vi "Populate Recorder List.vi"(4 "Seconds between samples":dbl=1.0 format="%_4f", 8 "error in (no error)":errorcluster, 11 "VISA Resourse Names":refnum<visa-resource-name>[](array[refnum])) -> (0 "error out":errorcluster, 2 "Names":string[](array[string]), 3 "Instrument List":refnum<class "Instrument Actor.lvclass">[](array[class]))   [LabVIEW 2019]
uses:
  Instrument Actor/Instrument Actor.lvclass
  NHMFL_Core/Libraries/Instruments/Device/Device type.ctl
  Temperature Controller/Temperature Controller.lvclass
  C:/GitHub/LabActor/Instrument Actor/Instrument Actor.lvclass
  NHMFL_Core/Libraries/Instruments/Cryo-con/Cryo-Con Driver/Cryo-Con Driver.lvclass
  C:/GitHub/NHMFL_Core/Libraries/Instruments/VISA Instrument/VISA Instrument.lvclass
  C:/GitHub/NHMFL_Core/Libraries/Instruments/Instrument Driver/Instrument Driver.lvclass
  C:/GitHub/NHMFL_Core/Libraries/Instruments/Temperature Controller Driver/Temperature Controller Driver.lvclass
  NHMFL_Core/Libraries/Instruments/VISA Instrument/VISA Instrument.lvclass/VISA Instrument.ctl
  NHMFL_Core/Libraries/Instruments/Instrument Driver/Instrument Driver.lvclass/Instrument Driver.ctl
  NHMFL_Core/Libraries/Instruments/Neocera/Neocera Driver/Neocera Driver.lvclass
  NHMFL_Core/Libraries/Instruments/LakeShore/LakeShore T Controller Driver/LakeShore T Controller Driver.lvclass
  NHMFL_Core/Libraries/Instruments/Arduino Temperature Controller/Arduino Temperature Controller Driver/Arduino Temperature Controller Driver.lvclass
  Channel Scanner/Channel Scanner.lvclass
  NHMFL_Core/Libraries/Instruments/LR-700/LR-700 Driver/LR-700 Driver.lvclass
  Instrument Actor/Instrument Actor.lvclass/Instrument Actor.ctl
  NHMFL_Core/Libraries/Instruments/Fluke/Fluke 1586A Driver.lvclass
  Fluke/Fluke Recorder.lvclass
  NHMFL_Core/Libraries/Instruments/Oxford/Oxford PS Driver/Oxford PS Driver.lvclass
  NHMFL_Core/Libraries/Instruments/AH/Andeen-Hagerling Driver/Andeen-Hagerling Driver.lvclass
  NHMFL_Core/Libraries/Instruments/Keithley/Keithley Driver/Keithley Driver.lvclass
  Keithley/Keithley Recorder.lvclass
  NHMFL_Core/Libraries/Instruments/Keithley/Keithley Driver/Keithley Driver.lvclass/Keithley Driver.ctl
  NHMFL_Core/Libraries/Instruments/LakeShore/LakeShore 370 Driver/LakeShore 370 Driver.lvclass
  NHMFL_Core/Libraries/Instruments/SRS/SRS Lockin Driver/SRS Lockin Driver.lvclass
  NHMFL_Core/Libraries/Instruments/HP/HP Counter Driver/HP Counter Driver.lvclass
  NHMFL_Core/Libraries/Instruments/Oxford/IPS120/IPS120.lvclass
  Sweeper/Sweeper.lvclass
  NHMFL_Core/Libraries/Instruments/Oxford/ITC503/ITC-503 Driver.lvclass
  NHMFL_Core/Libraries/Instruments/VISA Instrument/Write VISA resource.vi
  NHMFL_Core/Libraries/Instruments/Instrument Driver/Write Recorder name.vi
  Instrument Actor/Write Instrument driver.vi
  NHMFL_Core/Libraries/Instruments/Keithley/Keithley Driver/Write Source-meter.vi
  NHMFL_Core/Libraries/Instruments/Keithley/Keithley Driver/Write Auto-init.vi
  Temperature Controller/Write T ctl driver.vi
panel:
  in  "Instrument":T1=enum."LkShr 340 chA&B"
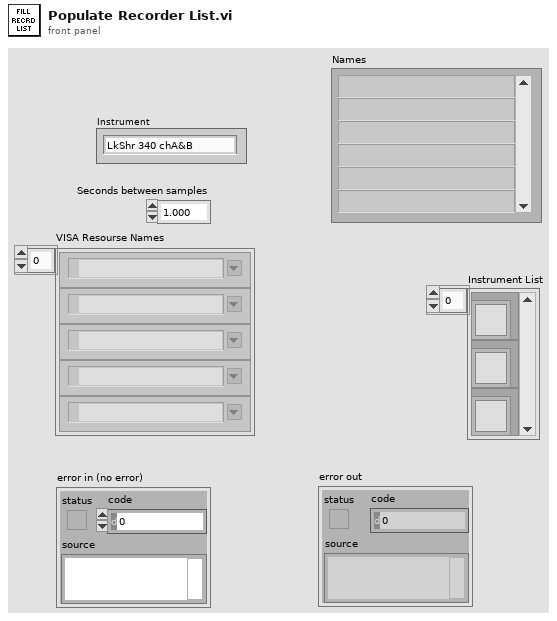
[diagram p1: front panel]
types:
  T1 = typedef "Device type.ctl" = enum16{"NONE", "Neocera 21", "LakeShore 335", "LakeShore 336", "LakeShore 340", "LkShr 340 chA&B", "LakeShore 370", "SRS 850", "SRS 830", "LR 700", "EG&G 5302", "EG&G 7260", "EG&G 7280", "AH 2500", "AH 2550", "AH 2700", "Keithley meter", "Keithley electrometer", "Keithley 182", "HP 5385", "HP 53181", "HP 53132", "ITC503", "IPS120", "Oxford Mercury IPS", "Oxford PS", "Test", "DC Facility Magnet", "Cryomagnetics PS", "Keithley 2400", "Keithley current source", "Cryo-Con 22C", "HP87NN", "HP4395A", "Agilent 34410A", "Arduino TC", "Cryo-Con 54", "Fluke 1586A"}
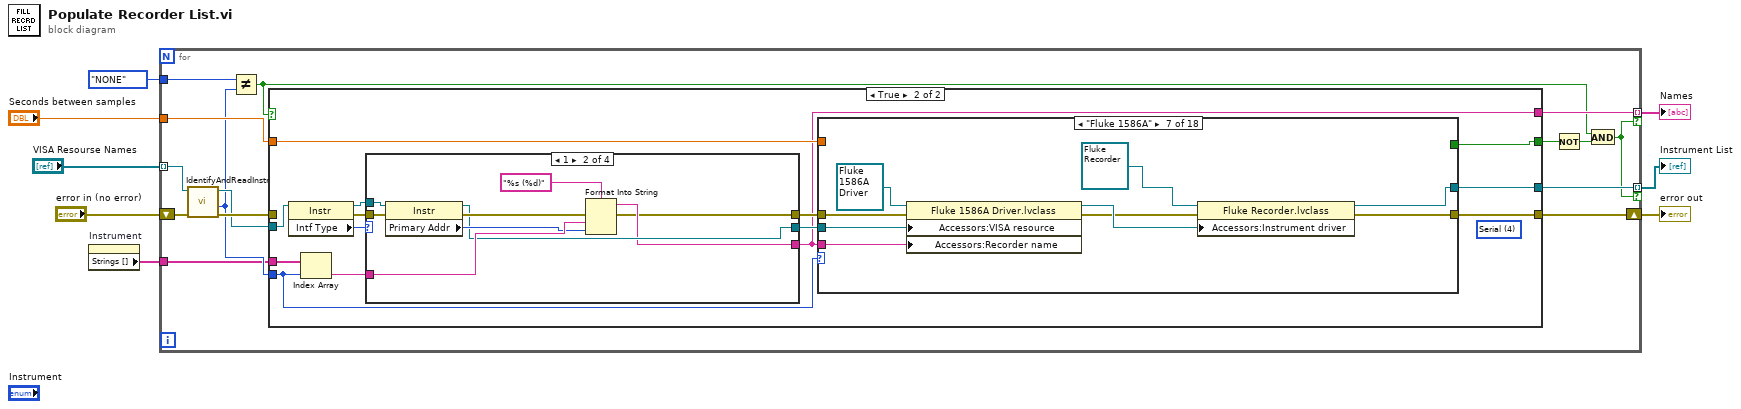
[diagram p0: block diagram]
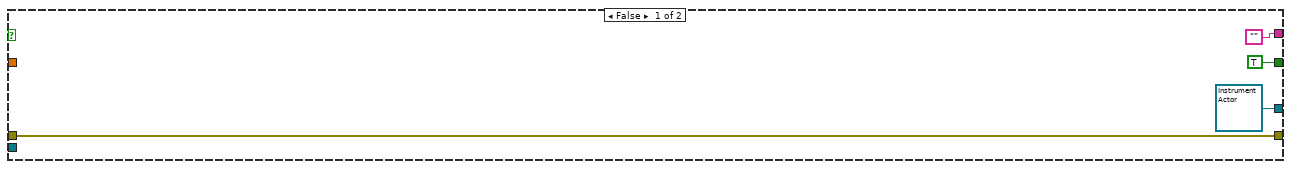
[diagram p2: hidden frame]
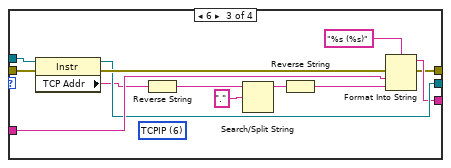
[diagram p4: hidden frame]
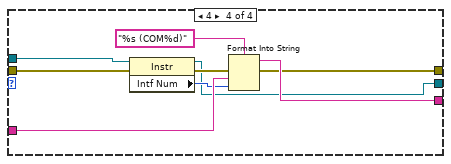
[diagram p5: hidden frame]
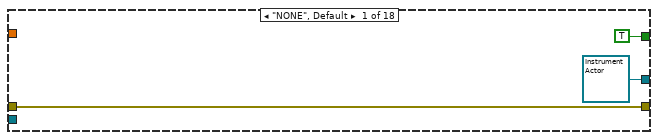
[diagram p6: hidden frame]
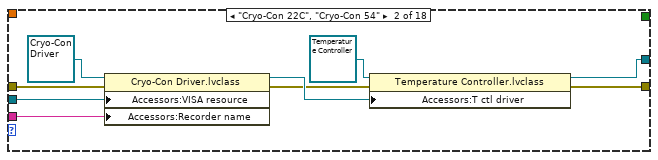
[diagram p7: hidden frame]
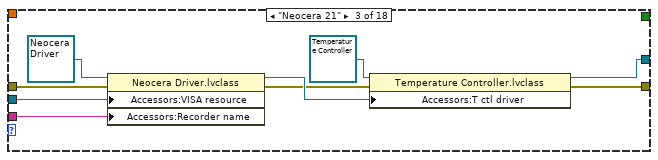
[diagram p8: hidden frame]
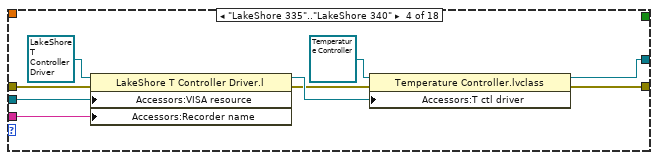
[diagram p9: hidden frame]
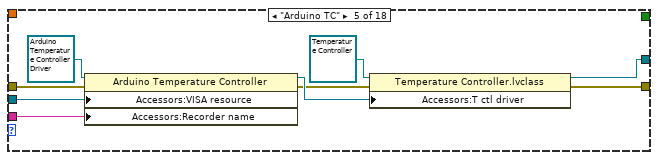
[diagram p10: hidden frame]
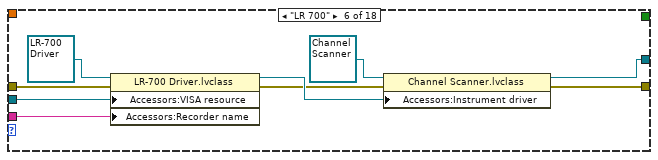
[diagram p11: hidden frame]
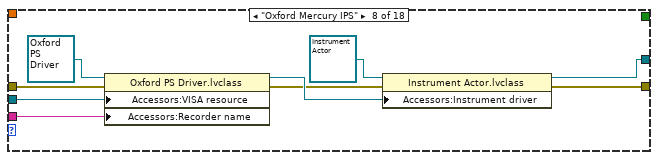
[diagram p12: hidden frame]
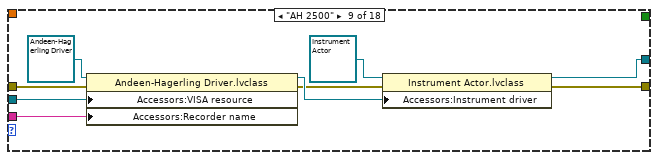
[diagram p13: hidden frame]
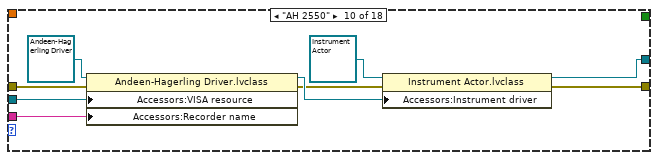
[diagram p14: hidden frame]
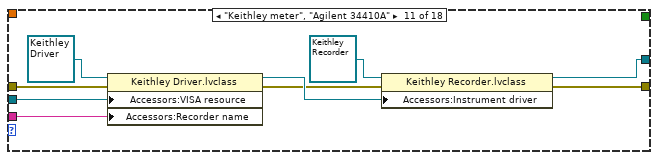
[diagram p15: hidden frame]
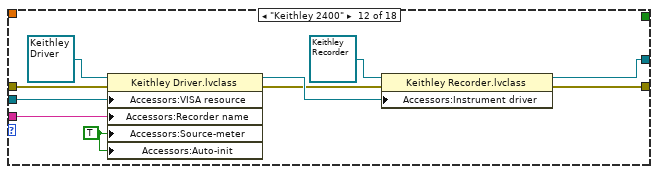
[diagram p16: hidden frame]
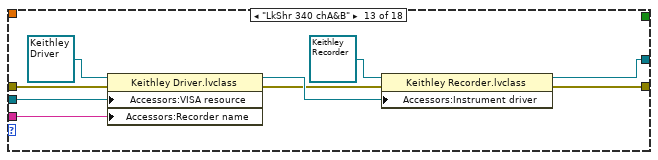
[diagram p17: hidden frame]
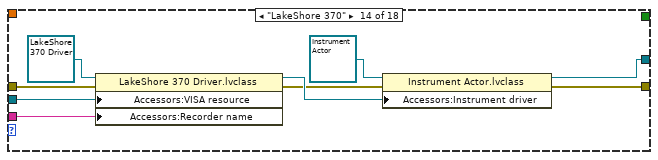
[diagram p18: hidden frame]
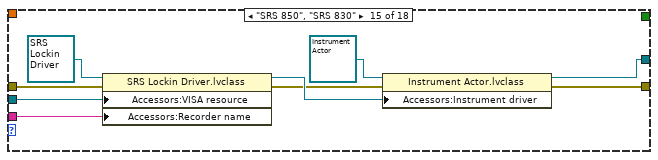
[diagram p19: hidden frame]
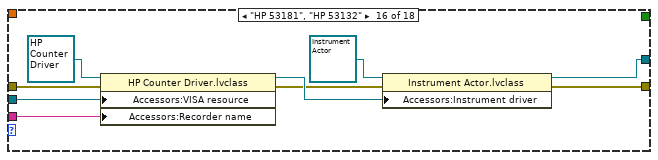
[diagram p20: hidden frame]
diagram:
  n1 = property on="Instrument" class="Enum (strict)"() -> ("Strings []"=w4:string[])  [unwired: 2 in, 2 out]
  n2 = for {
    tunnel: "VISA Resourse Names" -> [w21] mode=indexing
    shift-right: [w18] -> w6
    shift-left: "error in (no error)" -> [w23]
    tunnel: "Seconds between samples" -> [w20]
    tunnel: w4 -> [w15]
    tunnel: Device_type."NONE" ("Instrument") -> [w17]
    tunnel: [w14] -> w2 mode=indexing if=w11
    tunnel: [w13] -> w1 mode=indexing if=w11
    n3 = call "IdentifyAndReadInstr.vi"("error in (no error)"=w23, "VISA Resource Name"=w21) -> ("error out"=w22:errorcluster, "Instrument"=w16:T1, "VISA Resource Name Out"=w19:refnum<visa-resource-name>)  [unwired: 6 in, 1 out]
    n4 = Not Equal?(x=w17, y=w16) -> (x != y?=w12:bool)
    n5 = case shown="True" w12 {
      tunnel: w22 -> [w27 _]
      tunnel: w20 -> [_ w41]
      tunnel: w19 -> [_ w36]
      tunnel: w16 -> [_ w38]
      tunnel: [refnum<class "Instrument Actor.lvclass"> refnum ("Instrument Recorder.lvclass") w33] -> w14
      tunnel: [w27 w30] -> w18
      tunnel: w15 -> [_ w40]
      tunnel: ["" w29] -> w13
      tunnel: [TRUE w28] -> w10
      frame False {
      }
      frame True {
        (unwired) u16 4 items=["GPIB"=1, "VXI"=2, "GPIB-VXI"=3, "Serial"=4, "PXI"=5, "TCPIP"=6, "USB"=7, "FireWire"=9] ("Interface Information:Interface Type")
        n6 = property class="Instr"(reference=w36) -> (reference out=w37:refnum<visa-resource-name>, error out=w35:errorcluster, "Intf Type"=w34:u16)  [unwired: 1 in]
        n7 = Index Array(array=w40, index=w38) -> (element=w39:string)
        n8 = case shown="1" w34 {
          tunnel: w39 -> [w42 w51 w64 w73]
          tunnel: [w43 w49 w63 w67] -> w31
          tunnel: [w42 w48 w62 w71] -> w29
          tunnel: [w44 w47 w61 w70] -> w32
          tunnel: w37 -> [w43 w46 w60 w69]
          tunnel: w35 -> [w44 w45 w59 w68]
          frame 0, Default {
          }
          frame 1 {
            n9 = property class="Instr"(reference=w46, error in=w45) -> (reference out=w49:refnum<visa-resource-name>, error out=w53:errorcluster, "Primary Addr"=w50:u16)
            n10 = Format Into String(format string="%s (%d)", error in=w53, w51, w50) -> (resulting string=w48:string, error out=w47:errorcluster)  [unwired: 1 in]
          }
          frame 6 {
            (unwired) u16 6 items=["GPIB"=1, "VXI"=2, "GPIB-VXI"=3, "Serial"=4, "PXI"=5, "TCPIP"=6, "USB"=7, "FireWire"=9] ("Interface Information:Interface Type")
            n11 = property class="Instr"(reference=w60, error in=w59) -> (reference out=w63:refnum<visa-resource-name>, error out=w66:errorcluster, "TCP Addr"=w58:string)
            n12 = Reverse String(1:w58) -> (0:w56:string)
            n13 = Search/Split String(string=w56, search string/char (-)="." ("regular expression")) -> (substring before match=w55:string)  [unwired: 1 in, 2 out]
            n14 = Reverse String(1:w55) -> (0:w57:string)
            n15 = Format Into String(format string="%s (%s)", error in=w66, w64, w57) -> (resulting string=w62:string, error out=w61:errorcluster)  [unwired: 1 in]
          }
          frame 4 {
            n16 = property class="Instr"(reference=w69, error in=w68) -> (reference out=w67:refnum<visa-resource-name>, error out=w75:errorcluster, "Intf Num"=w72:u16)
            n17 = Format Into String(format string="%s (COM%d)", error in=w75, w73, w72) -> (resulting string=w71:string, error out=w70:errorcluster)  [unwired: 1 in]
          }
        }
        n18 = case shown="\"Fluke 1586A\"" w38 {
          tunnel: w32 -> [w78 w81 w90 w99 w108 w117 w127 w136 w145 w154 w163 w173 w182 w191 w200 w209 w219 w228]
          tunnel: [w78 w80 w89 w98 w107 w116 w126 w135 w144 w153 w162 w172 w181 w190 w199 w208 w218 w227] -> w30
          tunnel: [refnum<class "Instrument Actor.lvclass"> refnum ("Instrument Recorder.lvclass") w86 w95 w104 w113 w119 w129 w138 w147 w156 w165 w175 w184 w193 w202 w211 w221 w230] -> w33
          tunnel: w41 -> [_ _ _ _ _ _ _ _ _ _ _ _ _ _ _ _ _ _]
          tunnel: w31 -> [_ w83 w92 w101 w110 w121 w130 w139 w148 w157 w166 w176 w185 w194 w203 w212 w222 w231]
          tunnel: w29 -> [_ w79 w88 w97 w106 w115 w125 w134 w143 w152 w161 w171 w180 w189 w198 w207 w217 w226]
          tunnel: [TRUE _ _ _ _ _ _ _ _ _ _ _ _ _ _ _ _ _] -> w28
          frame "NONE", Default {
          }
          frame "Cryo-Con 22C", "Cryo-Con 54" {
            n19 = property class="Cryo-Con Driver.lvclass"(reference=refnum<class "Cryo-Con Driver.lvclass"> refnum ("Cryo-Con Driver.lvclass"), error in=w81, "Accessors:VISA resource"=w83, "Accessors:Recorder name"=w79) -> (reference out=w84:refnum<class "Cryo-Con Driver.lvclass">, error out=w82:errorcluster)
            n20 = property class="Temperature Controller.lvclass"(reference=refnum<class "Temperature Controller.lvclass"> refnum ("Temperature Controller.lvclass"), error in=w82, "Accessors:T ctl driver"=w84) -> (reference out=w86:refnum<class "Temperature Controller.lvclass">, error out=w80:errorcluster)
          }
          frame "Neocera 21" {
            n21 = property class="Neocera Driver.lvclass"(reference=refnum<class "Neocera Driver.lvclass"> refnum ("Neocera Driver.lvclass"), error in=w90, "Accessors:VISA resource"=w92, "Accessors:Recorder name"=w88) -> (reference out=w93:refnum<class "Neocera Driver.lvclass">, error out=w91:errorcluster)
            n22 = property class="Temperature Controller.lvclass"(reference=refnum<class "Temperature Controller.lvclass"> refnum ("Temperature Controller.lvclass"), error in=w91, "Accessors:T ctl driver"=w93) -> (reference out=w95:refnum<class "Temperature Controller.lvclass">, error out=w89:errorcluster)
          }
          frame "LakeShore 335".."LakeShore 340" {
            n23 = property class="LakeShore T Controller Driver.l"(reference=refnum<class "LakeShore T Controller Driver.lvclass"> refnum ("LakeShore T Controller Driver.lvclass"), error in=w99, "Accessors:VISA resource"=w101, "Accessors:Recorder name"=w97) -> (reference out=w102:refnum<class "LakeShore T Controller Driver.lvclass">, error out=w100:errorcluster)
            n24 = property class="Temperature Controller.lvclass"(reference=refnum<class "Temperature Controller.lvclass"> refnum ("Temperature Controller.lvclass"), error in=w100, "Accessors:T ctl driver"=w102) -> (reference out=w104:refnum<class "Temperature Controller.lvclass">, error out=w98:errorcluster)
          }
          frame "Arduino TC" {
            n25 = property class="Arduino Temperature Controller "(reference=refnum<class "Arduino Temperature Controller Driver.lvclass"> refnum ("Arduino Temperature Controller Driver.lvclass"), error in=w108, "Accessors:VISA resource"=w110, "Accessors:Recorder name"=w106) -> (reference out=w111:refnum<class "Arduino Temperature Controller Driver.lvclass">, error out=w109:errorcluster)
            n26 = property class="Temperature Controller.lvclass"(reference=refnum<class "Temperature Controller.lvclass"> refnum ("Temperature Controller.lvclass"), error in=w109, "Accessors:T ctl driver"=w111) -> (reference out=w113:refnum<class "Temperature Controller.lvclass">, error out=w107:errorcluster)
          }
          frame "LR 700" {
            n27 = property class="LR-700 Driver.lvclass"(reference=refnum<class "LR-700 Driver.lvclass"> refnum ("LR-700 Driver.lvclass"), error in=w117, "Accessors:VISA resource"=w121, "Accessors:Recorder name"=w115) -> (reference out=w122:refnum<class "LR-700 Driver.lvclass">, error out=w118:errorcluster)
            n28 = property class="Channel Scanner.lvclass"(reference=refnum<class "Channel Scanner.lvclass"> refnum ("Channel Scanner.lvclass"), error in=w118, "Accessors:Instrument driver"=w122) -> (reference out=w119:refnum<class "Channel Scanner.lvclass">, error out=w116:errorcluster)
          }
          frame "Fluke 1586A" {
            n29 = property class="Fluke 1586A Driver.lvclass"(reference=refnum<class "Fluke 1586A Driver.lvclass"> refnum ("Fluke 1586A Driver.lvclass"), error in=w127, "Accessors:VISA resource"=w130, "Accessors:Recorder name"=w125) -> (reference out=w131:refnum<class "Fluke 1586A Driver.lvclass">, error out=w128:errorcluster)
            n30 = property class="Fluke Recorder.lvclass"(reference=refnum<class "Fluke Recorder.lvclass"> refnum ("Instrument Recorder.lvclass"), error in=w128, "Accessors:Instrument driver"=w131) -> (reference out=w129:refnum<class "Fluke Recorder.lvclass">, error out=w126:errorcluster)
          }
          frame "Oxford Mercury IPS" {
            n31 = property class="Oxford PS Driver.lvclass"(reference=refnum<class "Oxford PS Driver.lvclass"> refnum ("Oxford PS Driver.lvclass"), error in=w136, "Accessors:VISA resource"=w139, "Accessors:Recorder name"=w134) -> (reference out=w140:refnum<class "Oxford PS Driver.lvclass">, error out=w137:errorcluster)
            n32 = property class="Instrument Actor.lvclass"(reference=refnum<class "Instrument Actor.lvclass"> refnum ("Instrument Recorder.lvclass"), error in=w137, "Accessors:Instrument driver"=w140) -> (reference out=w138:refnum<class "Instrument Actor.lvclass">, error out=w135:errorcluster)
          }
          frame "AH 2500" {
            n33 = property class="Andeen-Hagerling Driver.lvclass"(reference=refnum<class "Andeen-Hagerling Driver.lvclass"> refnum ("Andeen-Hagerling Driver.lvclass"), error in=w145, "Accessors:VISA resource"=w148, "Accessors:Recorder name"=w143) -> (reference out=w149:refnum<class "Andeen-Hagerling Driver.lvclass">, error out=w146:errorcluster)
            n34 = property class="Instrument Actor.lvclass"(reference=refnum<class "Instrument Actor.lvclass"> refnum ("Instrument Recorder.lvclass"), error in=w146, "Accessors:Instrument driver"=w149) -> (reference out=w147:refnum<class "Instrument Actor.lvclass">, error out=w144:errorcluster)
          }
          frame "AH 2550" {
            n35 = property class="Andeen-Hagerling Driver.lvclass"(reference=refnum<class "Andeen-Hagerling Driver.lvclass"> refnum ("Andeen-Hagerling Driver.lvclass"), error in=w154, "Accessors:VISA resource"=w157, "Accessors:Recorder name"=w152) -> (reference out=w158:refnum<class "Andeen-Hagerling Driver.lvclass">, error out=w155:errorcluster)
            n36 = property class="Instrument Actor.lvclass"(reference=refnum<class "Instrument Actor.lvclass"> refnum ("Instrument Recorder.lvclass"), error in=w155, "Accessors:Instrument driver"=w158) -> (reference out=w156:refnum<class "Instrument Actor.lvclass">, error out=w153:errorcluster)
          }
          frame "Keithley meter", "Agilent 34410A" {
            n37 = property class="Keithley Driver.lvclass"(reference=refnum<class "Keithley Driver.lvclass"> refnum ("Keithley Driver.lvclass"), error in=w163, "Accessors:VISA resource"=w166, "Accessors:Recorder name"=w161) -> (reference out=w167:refnum<class "Keithley Driver.lvclass">, error out=w164:errorcluster)
            n38 = property class="Keithley Recorder.lvclass"(reference=refnum<class "Keithley Recorder.lvclass"> refnum ("Instrument Recorder.lvclass"), error in=w164, "Accessors:Instrument driver"=w167) -> (reference out=w165:refnum<class "Keithley Recorder.lvclass">, error out=w162:errorcluster)
          }
          frame "Keithley 2400" {
            w169 = TRUE ("Source-meter")
            n39 = property class="Keithley Driver.lvclass"(reference=refnum<class "Keithley Driver.lvclass"> refnum ("Keithley Driver.lvclass"), error in=w173, "Accessors:VISA resource"=w176, "Accessors:Recorder name"=w171, "Accessors:Source-meter"=w169, "Accessors:Auto-init"=w169) -> (reference out=w177:refnum<class "Keithley Driver.lvclass">, error out=w174:errorcluster)
            n40 = property class="Keithley Recorder.lvclass"(reference=refnum<class "Keithley Recorder.lvclass"> refnum ("Instrument Recorder.lvclass"), error in=w174, "Accessors:Instrument driver"=w177) -> (reference out=w175:refnum<class "Keithley Recorder.lvclass">, error out=w172:errorcluster)
          }
          frame "LkShr 340 chA&B" {
            n41 = property class="Keithley Driver.lvclass"(reference=refnum<class "Keithley Driver.lvclass"> refnum ("Keithley Driver.lvclass"), error in=w182, "Accessors:VISA resource"=w185, "Accessors:Recorder name"=w180) -> (reference out=w186:refnum<class "Keithley Driver.lvclass">, error out=w183:errorcluster)
            n42 = property class="Keithley Recorder.lvclass"(reference=refnum<class "Keithley Recorder.lvclass"> refnum ("Instrument Recorder.lvclass"), error in=w183, "Accessors:Instrument driver"=w186) -> (reference out=w184:refnum<class "Keithley Recorder.lvclass">, error out=w181:errorcluster)
          }
          frame "LakeShore 370" {
            n43 = property class="LakeShore 370 Driver.lvclass"(reference=refnum<class "LakeShore 370 Driver.lvclass"> refnum ("LakeShore 370 Driver.lvclass"), error in=w191, "Accessors:VISA resource"=w194, "Accessors:Recorder name"=w189) -> (reference out=w195:refnum<class "LakeShore 370 Driver.lvclass">, error out=w192:errorcluster)
            n44 = property class="Instrument Actor.lvclass"(reference=refnum<class "Instrument Actor.lvclass"> refnum ("Instrument Recorder.lvclass"), error in=w192, "Accessors:Instrument driver"=w195) -> (reference out=w193:refnum<class "Instrument Actor.lvclass">, error out=w190:errorcluster)
          }
          frame "SRS 850", "SRS 830" {
            n45 = property class="SRS Lockin Driver.lvclass"(reference=refnum<class "SRS Lockin Driver.lvclass"> refnum ("SRS Lockin Driver.lvclass"), error in=w200, "Accessors:VISA resource"=w203, "Accessors:Recorder name"=w198) -> (reference out=w204:refnum<class "SRS Lockin Driver.lvclass">, error out=w201:errorcluster)
            n46 = property class="Instrument Actor.lvclass"(reference=refnum<class "Instrument Actor.lvclass"> refnum ("Instrument Recorder.lvclass"), error in=w201, "Accessors:Instrument driver"=w204) -> (reference out=w202:refnum<class "Instrument Actor.lvclass">, error out=w199:errorcluster)
          }
          frame "HP 53181", "HP 53132" {
            n47 = property class="HP Counter Driver.lvclass"(reference=refnum<class "HP Counter Driver.lvclass"> refnum ("HP Counter Driver.lvclass"), error in=w209, "Accessors:VISA resource"=w212, "Accessors:Recorder name"=w207) -> (reference out=w213:refnum<class "HP Counter Driver.lvclass">, error out=w210:errorcluster)
            n48 = property class="Instrument Actor.lvclass"(reference=refnum<class "Instrument Actor.lvclass"> refnum ("Instrument Recorder.lvclass"), error in=w210, "Accessors:Instrument driver"=w213) -> (reference out=w211:refnum<class "Instrument Actor.lvclass">, error out=w208:errorcluster)
          }
          frame "IPS120" {
            n49 = property class="IPS120.lvclass"(reference=refnum<class "IPS120.lvclass"> refnum ("IPS120.lvclass"), error in=w219, "Accessors:VISA resource"=w222, "Accessors:Recorder name"=w217) -> (reference out=w223:refnum<class "IPS120.lvclass">, error out=w220:errorcluster)
            n50 = property class="Sweeper.lvclass"(reference=refnum<class "Sweeper.lvclass"> refnum ("Sweeper.lvclass"), error in=w220, "Accessors:Instrument driver"=w223) -> (reference out=w221:refnum<class "Sweeper.lvclass">, error out=w218:errorcluster)
          }
          frame "ITC503" {
            n51 = property class="ITC-503 Driver.lvclass"(reference=refnum<class "ITC-503 Driver.lvclass"> refnum ("ITC-503 Driver.lvclass"), error in=w228, "Accessors:VISA resource"=w231, "Accessors:Recorder name"=w226) -> (reference out=w232:refnum<class "ITC-503 Driver.lvclass">, error out=w229:errorcluster)
            n52 = property class="Temperature Controller.lvclass"(reference=refnum<class "Temperature Controller.lvclass"> refnum ("Temperature Controller.lvclass"), error in=w229, "Accessors:Instrument driver"=w232) -> (reference out=w230:refnum<class "Temperature Controller.lvclass">, error out=w227:errorcluster)
          }
        }
      }
    }
    n53 = Not(x=w10) -> (.not. x?=w9:bool)
    n54 = And(x=w12, y=w9) -> (x .and. y?=w11:bool)
  }
  "error out" <- w6
  "Instrument List" <- w2
  "Names" <- w1
